vi "Calculadora.vi"() -> ()   [LabVIEW 2020]
uses:
  <vilib>/gmath/NI_Gmath.lvlib
panel:
  in  "E":bool
  in  "ANS":bool
  in  "Precicion":dbl
  in  "EXP":bool
  in  "Del":bool
  in  "In":bool
  in  "AC":bool
  in  "log":bool
  in  "sqrt(":bool
  in  "x2":bool
  in  "tan":bool
  in  "cos":bool
  in  "sin":bool
  in  "Pi":bool
  in  "(":bool
  in  ")":bool
  in  "Display":string
  in  "Punto":bool
  in  "=":bool
  in  "0":bool
  in  "9":bool
  in  "8":bool
  in  "7":bool
  in  "6":bool
  in  "5":bool
  in  "4":bool
  in  "3":bool
  in  "2":bool
  in  "1":bool
  in  "Divicion":bool
  in  "Multiplicacion":bool
  in  "Resta":bool
  in  "Suma":bool
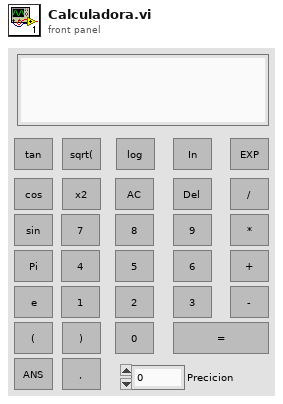
[diagram p1: front panel]
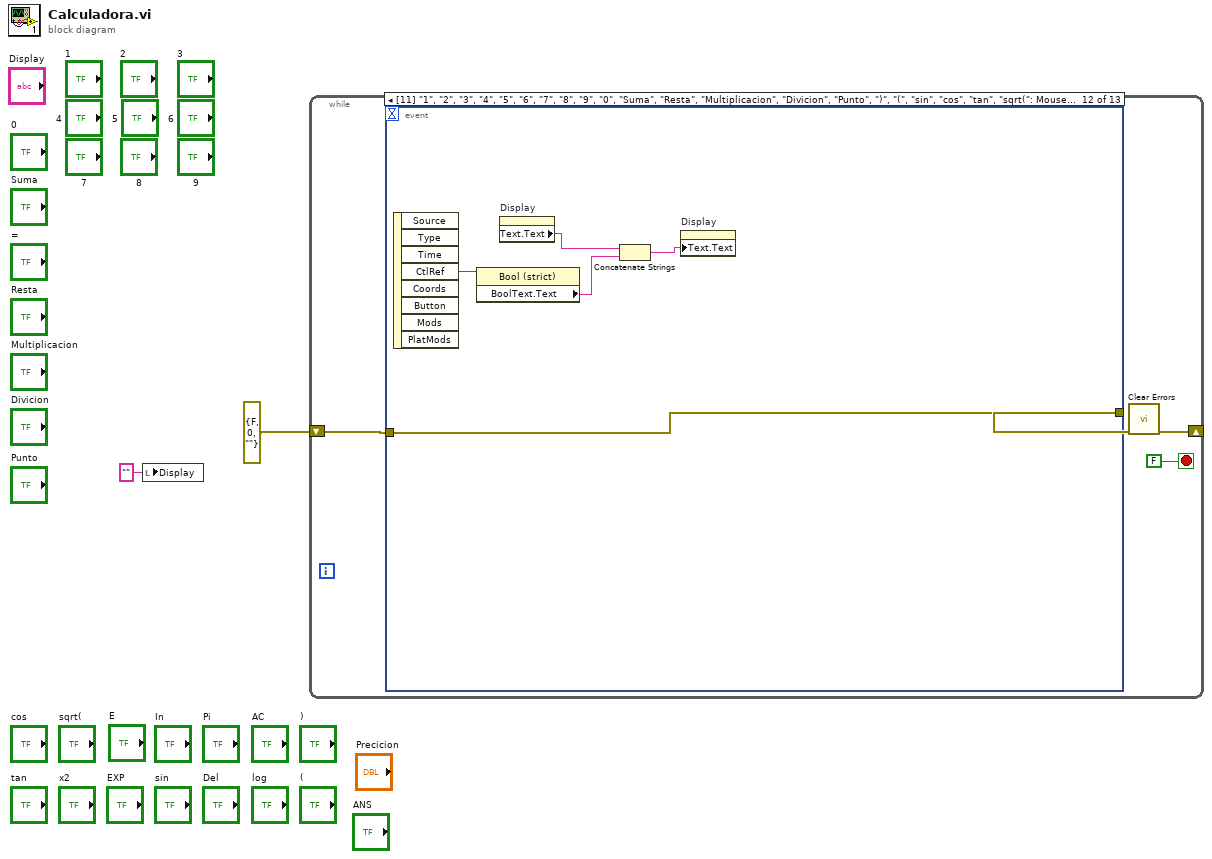
[diagram p0: block diagram]
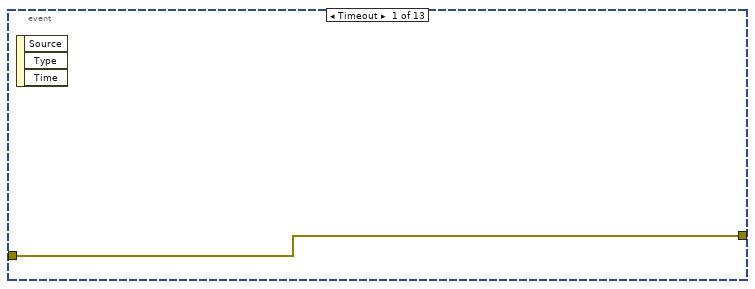
[diagram p2: hidden frame]
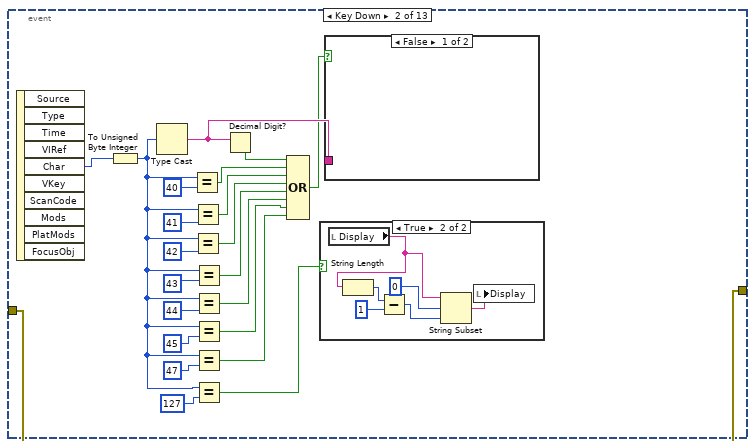
[diagram p3: hidden frame]
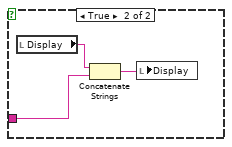
[diagram p5: hidden frame]
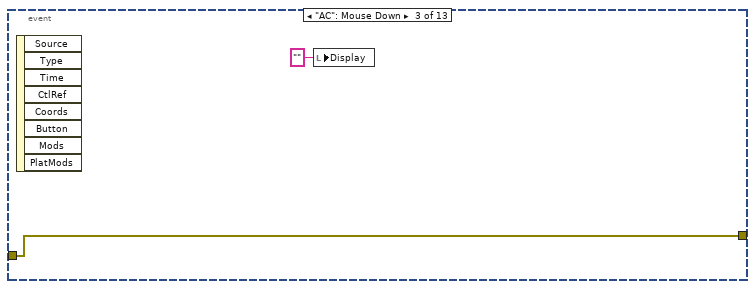
[diagram p6: hidden frame]
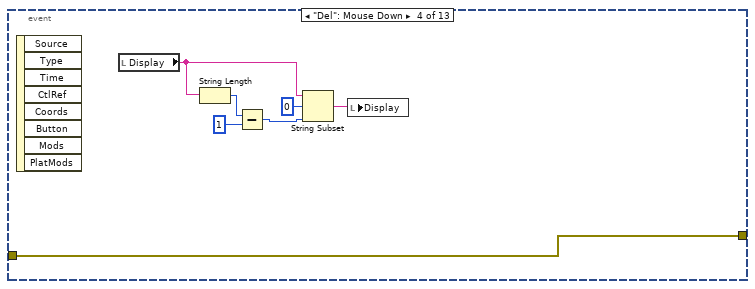
[diagram p7: hidden frame]
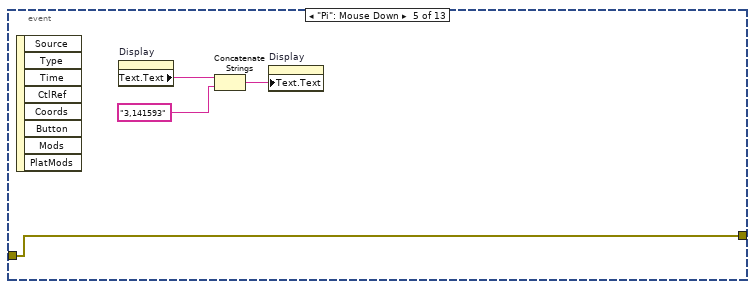
[diagram p8: hidden frame]
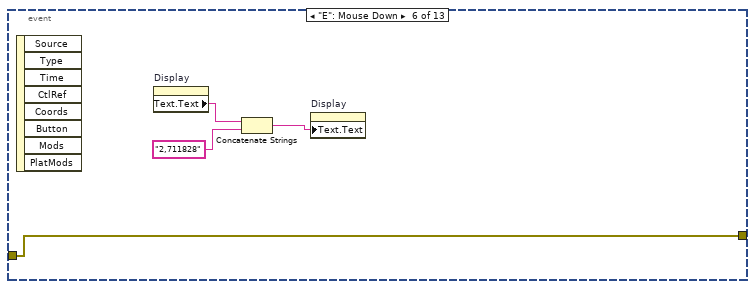
[diagram p9: hidden frame]
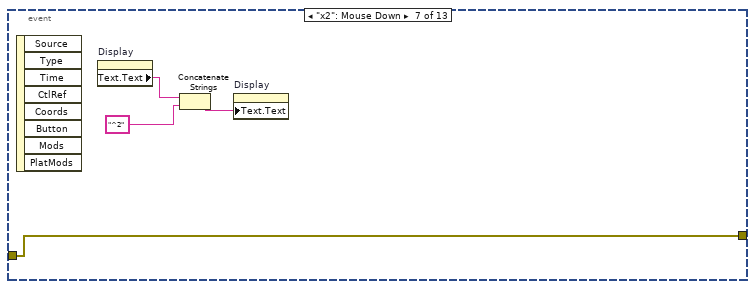
[diagram p10: hidden frame]
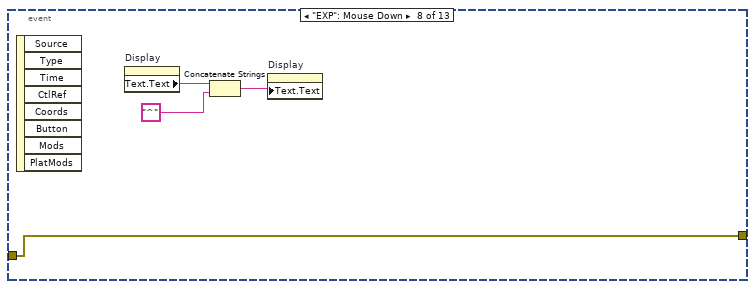
[diagram p11: hidden frame]
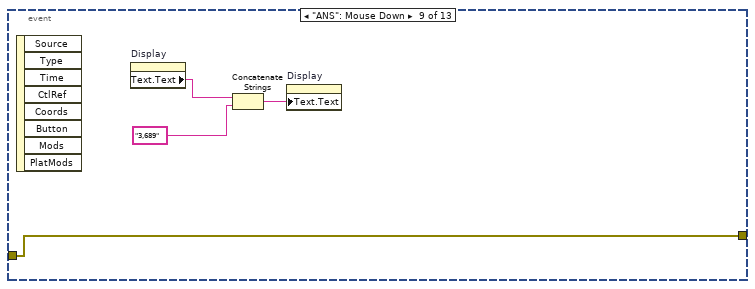
[diagram p12: hidden frame]
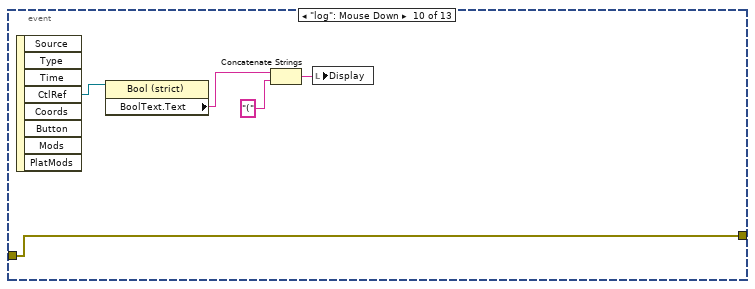
[diagram p13: hidden frame]
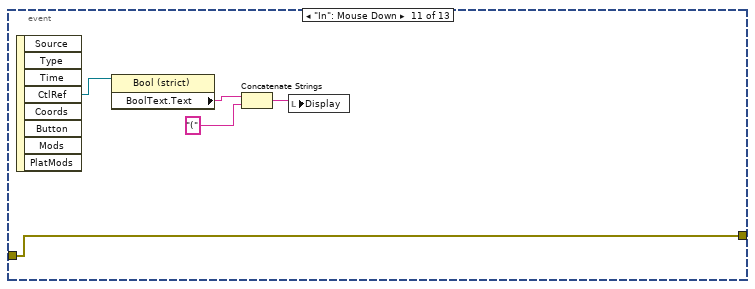
[diagram p14: hidden frame]
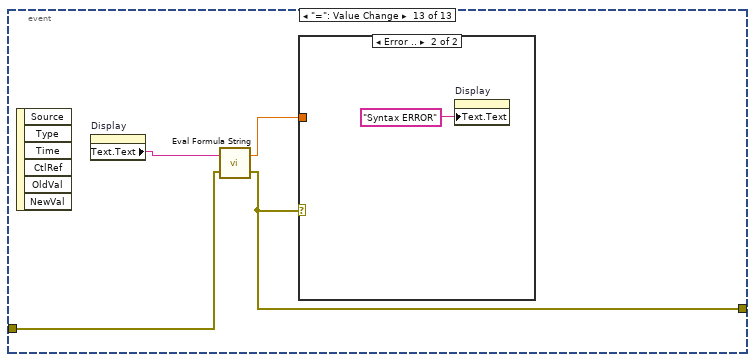
[diagram p15: hidden frame]
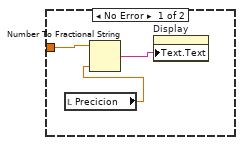
[diagram p16: hidden frame]
diagram:
  n1 = local write "Display"("" ("Display")) -> ()
  n2 = while {
    shift-right: [w4] -> _
    shift-left: errorcluster {"status"=FALSE, "code"=0, "source"=""} ("error in (no error)") -> [w6]
    stop <- FALSE stop-if-true
    n3 = event shown="[11] \"1\", \"2\", \"3\", \"4\", \"5\", \"6\", \"7\", \"8\", \"9\", \"0\", \"Suma\", \"Resta\", \"Multiplicacion\", \"Divicion\", \"Punto\", \")\", \"(\", \"sin\", \"cos\", \"tan\", \"sqrt(\": Mouse Down" {
      selector: _ -> [_ _ _ _ _ _ _ _ _ _ _ _ _]
      dyn-events: _ -> [_ _ _ _ _ _ _ _ _ _ _ _ _]
      timeout: _ -> [_ _ _ _ _ _ _ _ _ _ _ _ _]
      tunnel: w6 -> [w7 w9 w39 w47 w51 w52 w59 w62 w64 w72 w77 w80 w84]
      tunnel: [w7 w9 w39 w47 w51 w52 w59 w62 w64 w72 w77 w80 w83] -> w5
      event Timeout {
        n4 = event-data() -> ()  [unwired: 1 in, 3 out]
      }
      event Key Down {
        n5 = event-data() -> ("Char"=w29:i16)  [unwired: 1 in, 9 out]
        n6 = To Unsigned Byte Integer(number=w29) -> (unsigned 8bit integer=w8:u8)
        n7 = Type Cast(x=w8) -> (*(type *) &x=w28:string)  [unwired: 1 in]
        n8 = Equal?(x=w8, y=u8 40) -> (x = y?=w25:bool)
        n9 = Equal?(x=w8, y=u8 41) -> (x = y?=w23:bool)
        n10 = Equal?(x=w8, y=u8 42) -> (x = y?=w22:bool)
        n11 = Equal?(x=w8, y=u8 43) -> (x = y?=w21:bool)
        n12 = Equal?(x=w8, y=u8 44) -> (x = y?=w14:bool)
        n13 = Equal?(x=w8, y=u8 45) -> (x = y?=w13:bool)
        n14 = Equal?(x=w8, y=u8 47) -> (x = y?=w12:bool)
        n15 = Equal?(x=w8, y=127) -> (x = y?=w10:bool)
        n16 = Decimal Digit?(1:w28) -> (0:w26:bool)
        n17 = Compound Arithmetic op=OR(w26, w25, w23, w22, w21, w14, w13, w12) -> (w27:bool)
        n18 = case shown="True" w10 {
          frame False {
          }
          frame True {
            n19 = local read "Display"() -> (w30:string)
            n20 = String Length(string=w30) -> (length=w33:i32)
            n21 = Subtract(x=w33, y=1) -> (x-y=w34:i32)
            n22 = String Subset(string=w30, offset (0)=0, length (rest)=w34) -> (substring=w35:string)
            n23 = local write "Display"(w35) -> ()
          }
        }
        n24 = case shown="False" w27 {
          tunnel: w28 -> [_ w37]
          frame False {
          }
          frame True {
            n25 = local read "Display"() -> (w38:string)
            n26 = Concatenate Strings(w38, w37) -> (w36:string)
            n27 = local write "Display"(w36) -> ()
          }
        }
      }
      event "AC": Mouse Down {
        n28 = event-data() -> ()  [unwired: 1 in, 8 out]
        n29 = local write "Display"("" ("Display")) -> ()
      }
      event "Del": Mouse Down {
        n30 = event-data() -> ()  [unwired: 1 in, 8 out]
        n31 = local read "Display"() -> (w42:string)
        n32 = String Length(string=w42) -> (length=w46:i32)
        n33 = Subtract(x=w46, y=1) -> (x-y=w43:i32)
        n34 = String Subset(string=w42, offset (0)=0, length (rest)=w43) -> (substring=w41:string)
        n35 = local write "Display"(w41) -> ()
      }
      event "Pi": Mouse Down {
        n36 = event-data() -> ()  [unwired: 1 in, 8 out]
        n37 = property on="Display" class="Str"() -> ("Text.Text"=w49:string)  [unwired: 2 in, 2 out]
        n38 = Concatenate Strings(w49, "3,141593" ("Pi")) -> (w50:string)
        n39 = property on="Display" class="Str"("Text.Text"=w50) -> ()  [unwired: 2 in, 2 out]
      }
      event "E": Mouse Down {
        n40 = event-data() -> ()  [unwired: 1 in, 8 out]
        n41 = property on="Display" class="Str"() -> ("Text.Text"=w55:string)  [unwired: 2 in, 2 out]
        n42 = Concatenate Strings(w55, "2,711828" ("E")) -> (w54:string)
        n43 = property on="Display" class="Str"("Text.Text"=w54) -> ()  [unwired: 2 in, 2 out]
      }
      event "x2": Mouse Down {
        n44 = event-data() -> ()  [unwired: 1 in, 8 out]
        n45 = property on="Display" class="Str"() -> ("Text.Text"=w57:string)  [unwired: 2 in, 2 out]
        n46 = Concatenate Strings(w57, "^2" ("x2")) -> (w58:string)
        n47 = property on="Display" class="Str"("Text.Text"=w58) -> ()  [unwired: 2 in, 2 out]
      }
      event "EXP": Mouse Down {
        n48 = event-data() -> ()  [unwired: 1 in, 8 out]
        n49 = property on="Display" class="Str"() -> ("Text.Text"=w61:string)  [unwired: 2 in, 2 out]
        n50 = Concatenate Strings(w61, "^" ("EXP")) -> (w63:string)
        n51 = property on="Display" class="Str"("Text.Text"=w63) -> ()  [unwired: 2 in, 2 out]
      }
      event "ANS": Mouse Down {
        n52 = event-data() -> ()  [unwired: 1 in, 8 out]
        n53 = property on="Display" class="Str"() -> ("Text.Text"=w67:string)  [unwired: 2 in, 2 out]
        n54 = Concatenate Strings(w67, "3,689" ("ANS")) -> (w66:string)
        n55 = property on="Display" class="Str"("Text.Text"=w66) -> ()  [unwired: 2 in, 2 out]
      }
      event "log": Mouse Down {
        n56 = event-data() -> ("CtlRef"=w69:refnum<vi>)  [unwired: 1 in, 7 out]
        n57 = property class="Bool (strict)"(reference=w69) -> ("BoolText.Text"=w68:string)  [unwired: 1 in, 2 out]
        n58 = Concatenate Strings(w68, "(" ("Boolean Text.Text")) -> (w70:string)
        n59 = local write "Display"(w70) -> ()
      }
      event "In": Mouse Down {
        n60 = event-data() -> ("CtlRef"=w76:refnum<vi>)  [unwired: 1 in, 7 out]
        n61 = property class="Bool (strict)"(reference=w76) -> ("BoolText.Text"=w74:string)  [unwired: 1 in, 2 out]
        n62 = Concatenate Strings(w74, "(") -> (w73:string)
        n63 = local write "Display"(w73) -> ()
      }
      event "1", "2", "3", "4", "5", "6", "7", "8", "9", "0", "Suma", "Resta", "Multiplicacion", "Divicion", "Punto", ")", "(", "sin", "cos", "tan", "sqrt(": Mouse Down {
        n64 = event-data() -> ("CtlRef"=w82:refnum<vi>)  [unwired: 1 in, 7 out]
        n65 = property class="Bool (strict)"(reference=w82) -> ("BoolText.Text"=w81:string)  [unwired: 1 in, 2 out]
        n66 = property on="Display" class="Str"() -> ("Text.Text"=w79:string)  [unwired: 2 in, 2 out]
        n67 = Concatenate Strings(w79, w81) -> (w78:string)
        n68 = property on="Display" class="Str"("Text.Text"=w78) -> ()  [unwired: 2 in, 2 out]
      }
      event "=": Value Change {
        n69 = event-data() -> ()  [unwired: 1 in, 6 out]
        n70 = property on="Display" class="Str"() -> ("Text.Text"=w86:string)  [unwired: 2 in, 2 out]
        n71 = call <vilib>:"Eval Formula String.vi"("error in (no error)"=w84, "formula"=w86) -> ("error out"=w83:errorcluster, "y value"=w85:dbl)
        n72 = case shown="Error .." w83 {
          tunnel: w85 -> [w89 _]
          frame No Error {
            n73 = local read "Precicion"() -> (w87:dbl)
            n74 = Number To Fractional String(number=w89, precision (6)=w87) -> (F-format string=w88:string)  [unwired: 2 in]
            n75 = property on="Display" class="Str"("Text.Text"=w88) -> ()  [unwired: 2 in, 2 out]
          }
          frame Error {
            n76 = property on="Display" class="Str"("Text.Text"="Syntax ERROR" ("Value")) -> ()  [unwired: 2 in, 2 out]
          }
        }
      }
    }
    n77 = call <vilib>:"Clear Errors.vi"("error in (no error)"=w5) -> ("error out"=w4:errorcluster)  [unwired: 5 in, 1 out]
  }
